vi "XY Chart.vi"(11 "X":dbl[](array[numeric]) format="%0.2f") -> (0 "standard deviation":dbl format="%0.2f", 1 "mean":dbl format="%0.2f", 3 "XY Graph":T1(graph))   [LabVIEW 2009]
uses:
  <vilib>/Analysis/NI_AALPro.lvlib
  <vilib>/Analysis/NI_AALBase.lvlib
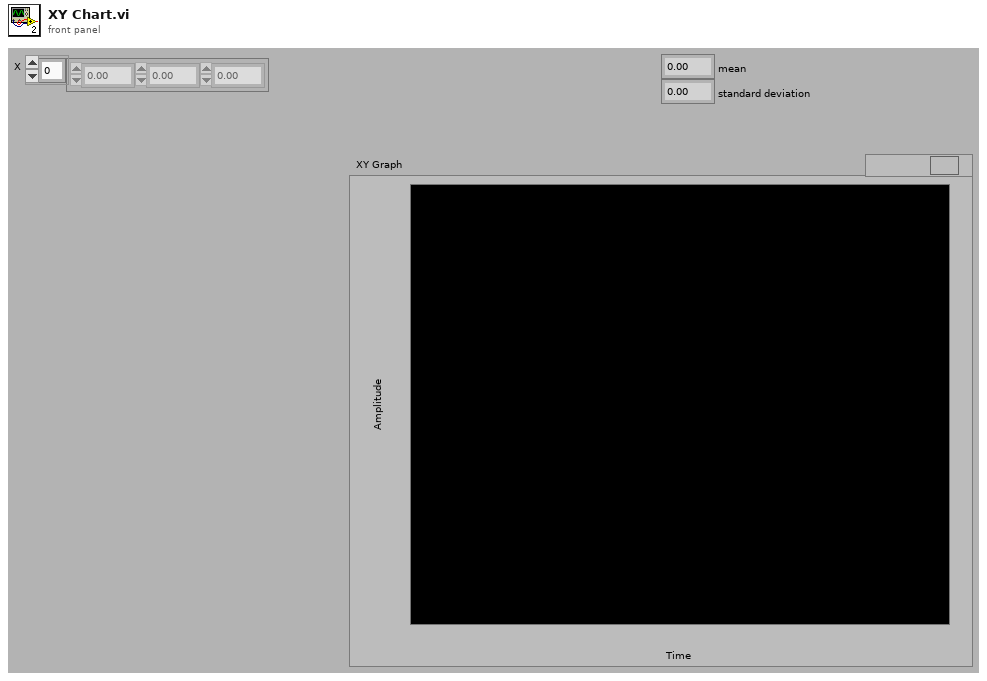
[diagram p1: front panel]
types:
  T1 = cluster{"X Values":dbl[], "Histogram: h(x)":i32[]}
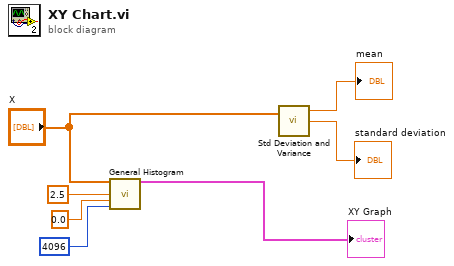
[diagram p0: block diagram]
diagram:
  n1 = call <vilib>:"General Histogram.vi"("X"="X", "max"=2.5, "min"=0.0, "# bins"=4096) -> ("Histogram Graph"=→"XY Graph":T1)  [unwired: 7 in, 4 out]
  n2 = call <vilib>:"Std Deviation and Variance.vi"("X"="X") -> ("mean"=→"mean":dbl, "standard deviation"=→"standard deviation":dbl)  [unwired: 1 in, 1 out]
